vi "TDMS GET DATA MULTI VALUES.vi"(5 "offset":i32, 7 "Grupo":string, 8 "error in":errorcluster, 10 "channel name(s) in":string, 11 "file path":path) -> (0 "error out":errorcluster, 2 "lengh":i32, 3 "transposed array":string[][](array[string]))   [LabVIEW 2015]
panel:
  out "data 2":timestamp[](array[timestamp])
  out "data":string[](array[string])
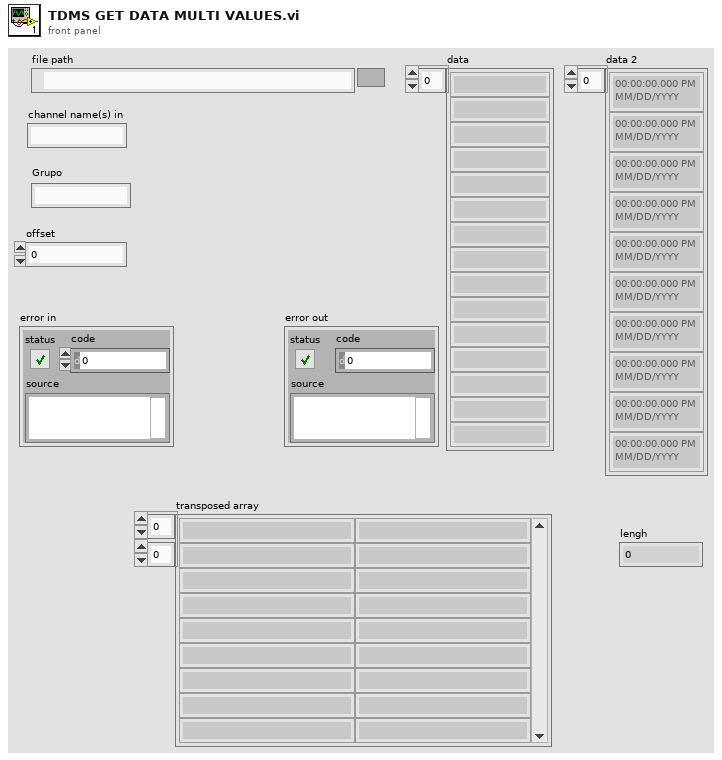
[diagram p1: front panel]
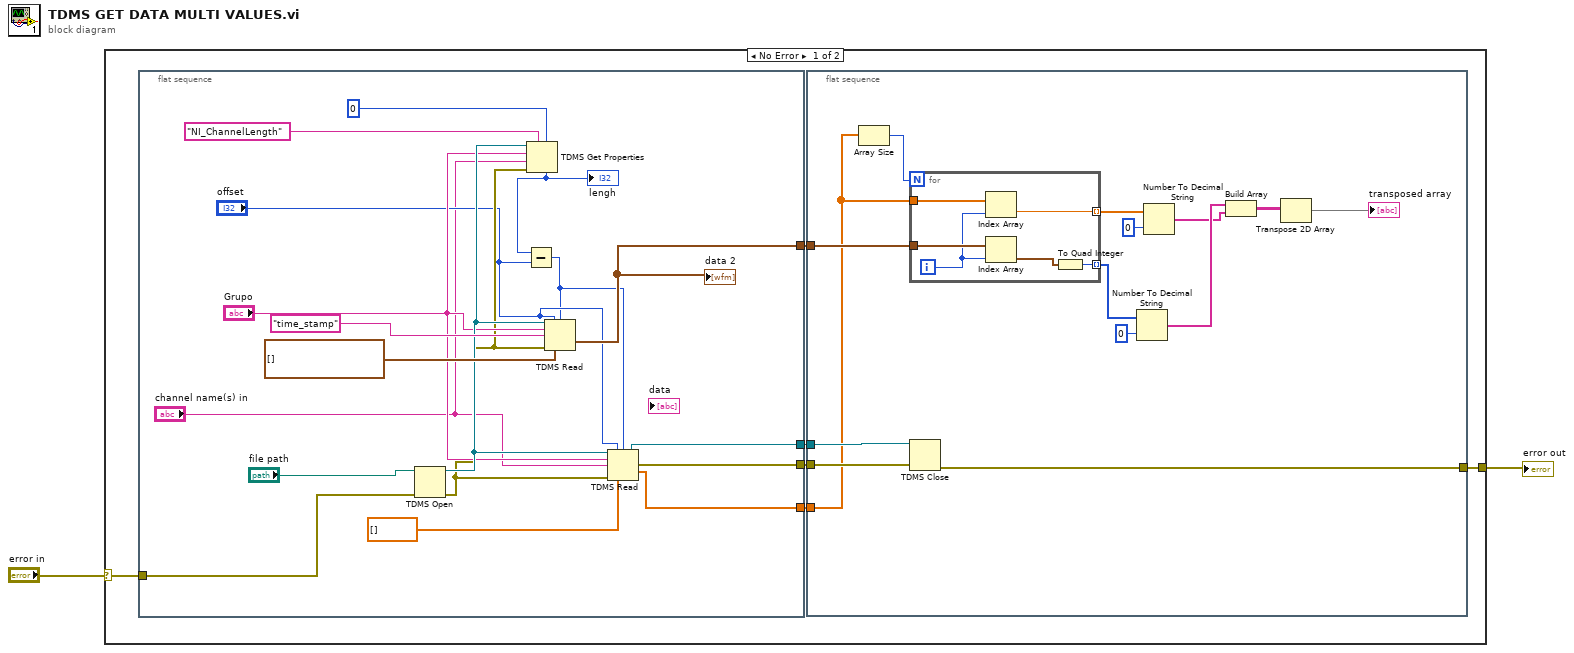
[diagram p0: block diagram]
diagram:
  n1 = case shown="No Error" "error in" {
    selector: "error in" -> [w3 w47]
    tunnel: [w4 w47] -> w2
    frame No Error {
      n2 = flat-sequence {
        tunnel: [w45] -> w8
        tunnel: [w44] -> w7
        tunnel: [w31] -> w6
        tunnel: [w35] -> w5
        tunnel: w3 -> [w29]
        frame #0 {
          n3 = TDMS Open(8:w29, 11:"file path") -> (0:w36:errorcluster, 3:w38:refnum<k34>)  [unwired: 5 in]
          n4 = TDMS Get Properties(5:0, 7:"NI_ChannelLength" ("property name"), 8:w36, 9:"channel name(s) in", 10:"Grupo", 11:w38) -> (4:w34:i32)  [unwired: 5 out]
          "lengh" <- w34
          n5 = Subtract(x=w34, y="offset") -> (x-y=w30:i32)
          n6 = TDMS Read(0:w38, 1:"offset", 2:w30, 5:"Grupo", 7:"time_stamp", 11:w36, 12:timestamp[] []) -> (10:w35:timestamp[])  [unwired: 1 in, 5 out]
          "data 2" <- w35
          n7 = TDMS Read(0:w38, 1:"offset", 2:w30, 5:"Grupo", 7:"channel name(s) in", 11:w36, 12:dbl[] []) -> (4:w45:refnum<k34>, 10:w31:dbl[], 15:w44:errorcluster)  [unwired: 1 in, 3 out]
        }
      }
      n8 = flat-sequence {
        tunnel: w8 -> [w22]
        tunnel: w7 -> [w21]
        tunnel: w6 -> [w13]
        tunnel: w5 -> [w20]
        tunnel: [w9] -> w4
        frame #0 {
          n9 = Array Size(array=w13) -> (size(s)=w18:i32)
          n10 = for {
            N: w18 -> [_]
            tunnel: w13 -> [w28]
            tunnel: w20 -> [w27]
            tunnel: [w25] -> w16 mode=indexing
            tunnel: [w23] -> w10 mode=indexing
            i -> [w26]
            n11 = Index Array(array=w28, index=w26) -> (element=w25:dbl)
            n12 = Index Array(array=w27, index=w26) -> (element=w24:timestamp)
            n13 = To Quad Integer(1:w24) -> (0:w23:i64)
          }
          n14 = TDMS Close(8:w21, 11:w22) -> (0:w9:errorcluster)  [unwired: 1 out]
          n15 = Number To Decimal String(number=w10, width (-)=i16 0) -> (decimal integer string=w19:string[])
          n16 = Number To Decimal String(number=w16, width (-)=i16 0) -> (decimal integer string=w15:string[])
          n17 = Build Array(w19, w15) -> (w11:string[][])
          n18 = Transpose 2D Array(2D array=w11) -> (transposed array=→"transposed array":string[][])
        }
      }
    }
    frame Error {
    }
  }
  "error out" <- w2
